vi "AudioStreamer.IsTriggered.vi"() -> (0 "triggered":bool)   [LabVIEW 2020]
uses:
  Typedefs/AudioStreamer.Globals.vi
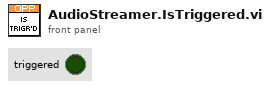
[diagram p1: front panel]
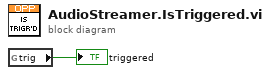
[diagram p0: block diagram]
diagram:
  n1 = global read "AudioStreamer.Globals.vi" "trig"() -> (→"triggered":bool)
